vi "Nichtlinearer Beobachter.vi"(0 "x1":dbl, 1 "x3":dbl, 2 "u":dbl) -> (20 "x1_":dbl, 21 "x2_":dbl, 22 "x3_":dbl, 23 "x4_":dbl, 24 "Differenz_x1":dbl)   [LabVIEW 2014]
uses:
  Root.vi
  Root1.vi
  d(f2+g2u)_dx3.vi
  d(f2+g2u)_dx4.vi
  d(f4+g4u)_dx3.vi
  d(f4+g4u)_dx4.vi
  f2+g2u.vi
  f4+g4u.vi
  <vilib>/Simulation/Implementation/Shared/SIMSCR Execution Mode.ctl
  <vilib>/Simulation/Scripting/Companion Diagram/SimConfigNode/SimParams.ctl
  <vilib>/Simulation/Scripting/Companion Diagram/SimConfigNode/_simSolvers.ctl
  <vilib>/Simulation/Param Hierarchy/Typedefs/SIMPH Param Control Actions.ctl
  <vilib>/Simulation/Implementation/Shared/SIM limit type.ctl
  <vilib>/Simulation/Implementation/Shared/NILVSim_ParamChanged.vi
  <vilib>/Simulation/Implementation/Shared/NILVSIM_BeginStep.vi
  <vilib>/Simulation/SignalArithmetic/Implementation/NILVSim Gain.llb/SIM Gain (scalar).vi
  <vilib>/Simulation/SignalDisplay/Implementation/NILVSim Time Waveform.llb/SIM Time Waveform (vector).vi
  <vilib>/Simulation/SignalDisplay/Implementation/NILVSim Time Waveform.llb/SIM Time Waveform (scalar).vi
  <vilib>/Simulation/Nonlinear/Implementation/NILVSim Saturation.llb/SIM Saturation (scalar).vi
  <vilib>/Simulation/ContinuousLinear/Implementation/NILVSim Integrator new.llb/SIM Integrator distributor (scalar).vi
  <vilib>/Simulation/ContinuousLinear/Implementation/NILVSim Integrator new.llb/SIM Integrator collector (scalar).vi
  <vilib>/Simulation/Implementation/Shared/NILVSim_Manager.vi
  <vilib>/Utility/error.llb/Clear Errors.vi
  <vilib>/Simulation/Implementation/Shared/NILVSim_FinalizeModel.vi
  <vilib>/Simulation/Implementation/Shared/SIM Unbundle Sim Info.vi
  <vilib>/Simulation/Implementation/Shared/SIMSH Read Queue.vi
  f24.vi
  f44.vi
  f23.vi
  x3_.vi
  diff_x3.vi
  L32.vi
  diff_x1.vi
  L31.vi
  L42.vi
  L41.vi
  L11.vi
  L21.vi
  F.vi
  x4_.vi
  f43.vi
  <vilib>/Simulation/Implementation/Shared/NILVSim_Initialize.vi
  <vilib>/Simulation/Utility/Implementation/NILVSim Get Time and IsAcceptedStep.vi
  <vilib>/Simulation/Implementation/Shared/NILVSim_GetModelError.vi
  <vilib>/Simulation/Implementation/Shared/SIM SimErrorHandler.vi
  <vilib>/Simulation/Implementation/Shared/SIM Bundle Sim Info.vi
  <vilib>/Simulation/Scripting/Companion Diagram/SimConfigNode/SimDog.xnode
  <vilib>/Simulation/Implementation/XNodeFramework/SimXNode/SimX.xnode
  <vilib>/Simulation/ContinuousLinear/Implementation/NILVSim Integrator new.llb/SIM Integrator (scalar).vi
  <vilib>/Simulation/Implementation/Shared/NI_SIM_Implementation.lvlib
panel:
  out "Scope9":waveform(dbl)[](graph)
  out "Scope8":waveform(dbl)(graph)
  out "Scope7":waveform(dbl)(graph)
  out "Scope6":waveform(dbl)[](graph)
  out "Scope5":waveform(dbl)(graph)
  out "Scope4":waveform(dbl)[](graph)
  out "Scope3":waveform(dbl)[](graph)
  out "Scope2":waveform(dbl)(graph)
  out "Scope1":waveform(dbl)(graph)
  out "Scope":waveform(dbl)(graph)
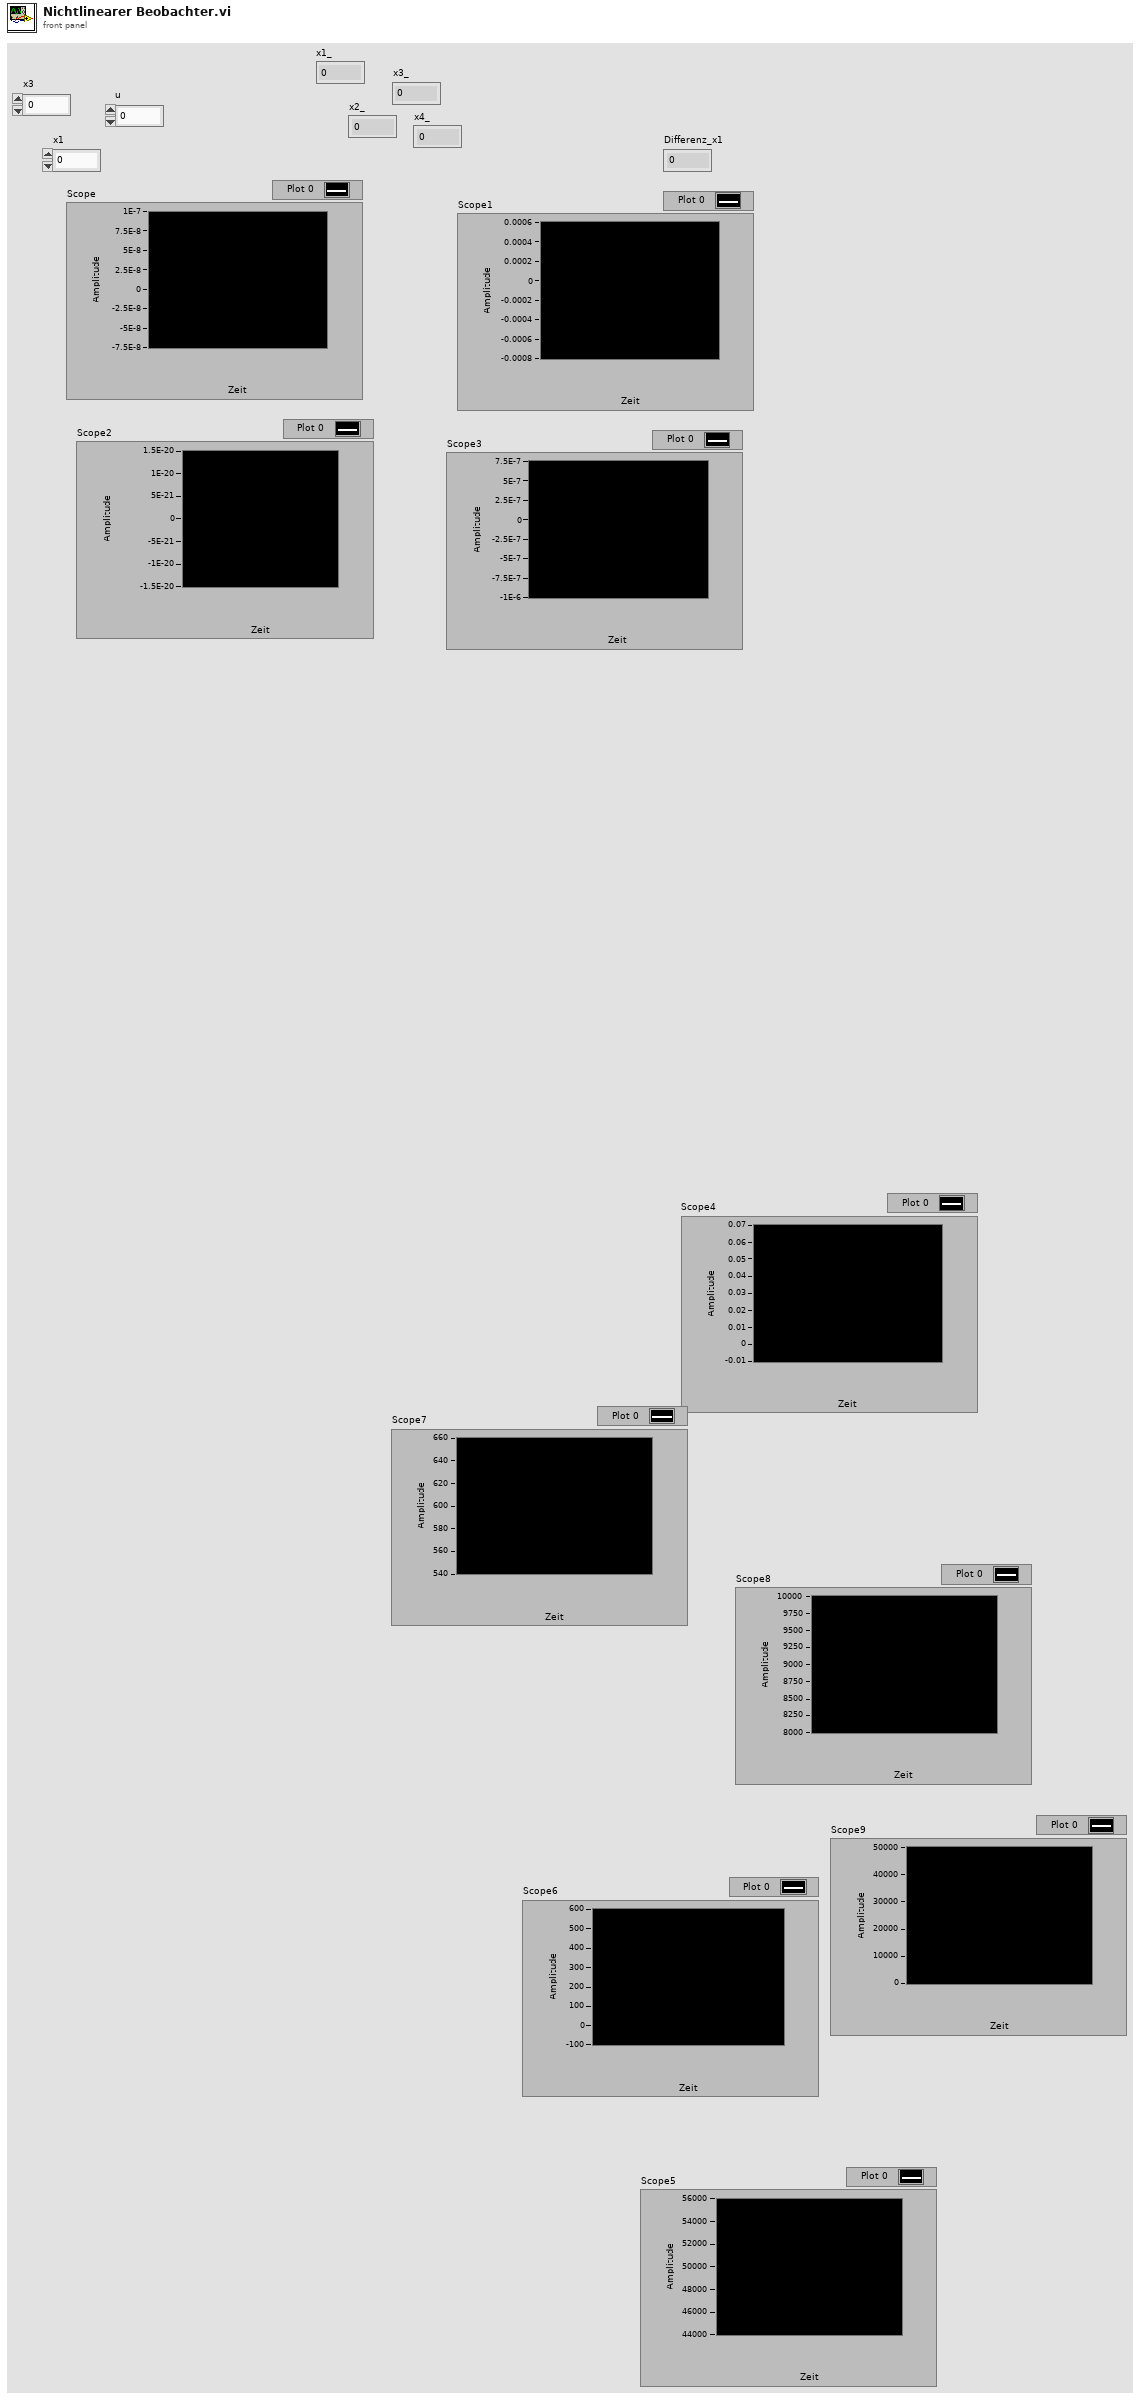
[diagram p1: front panel]
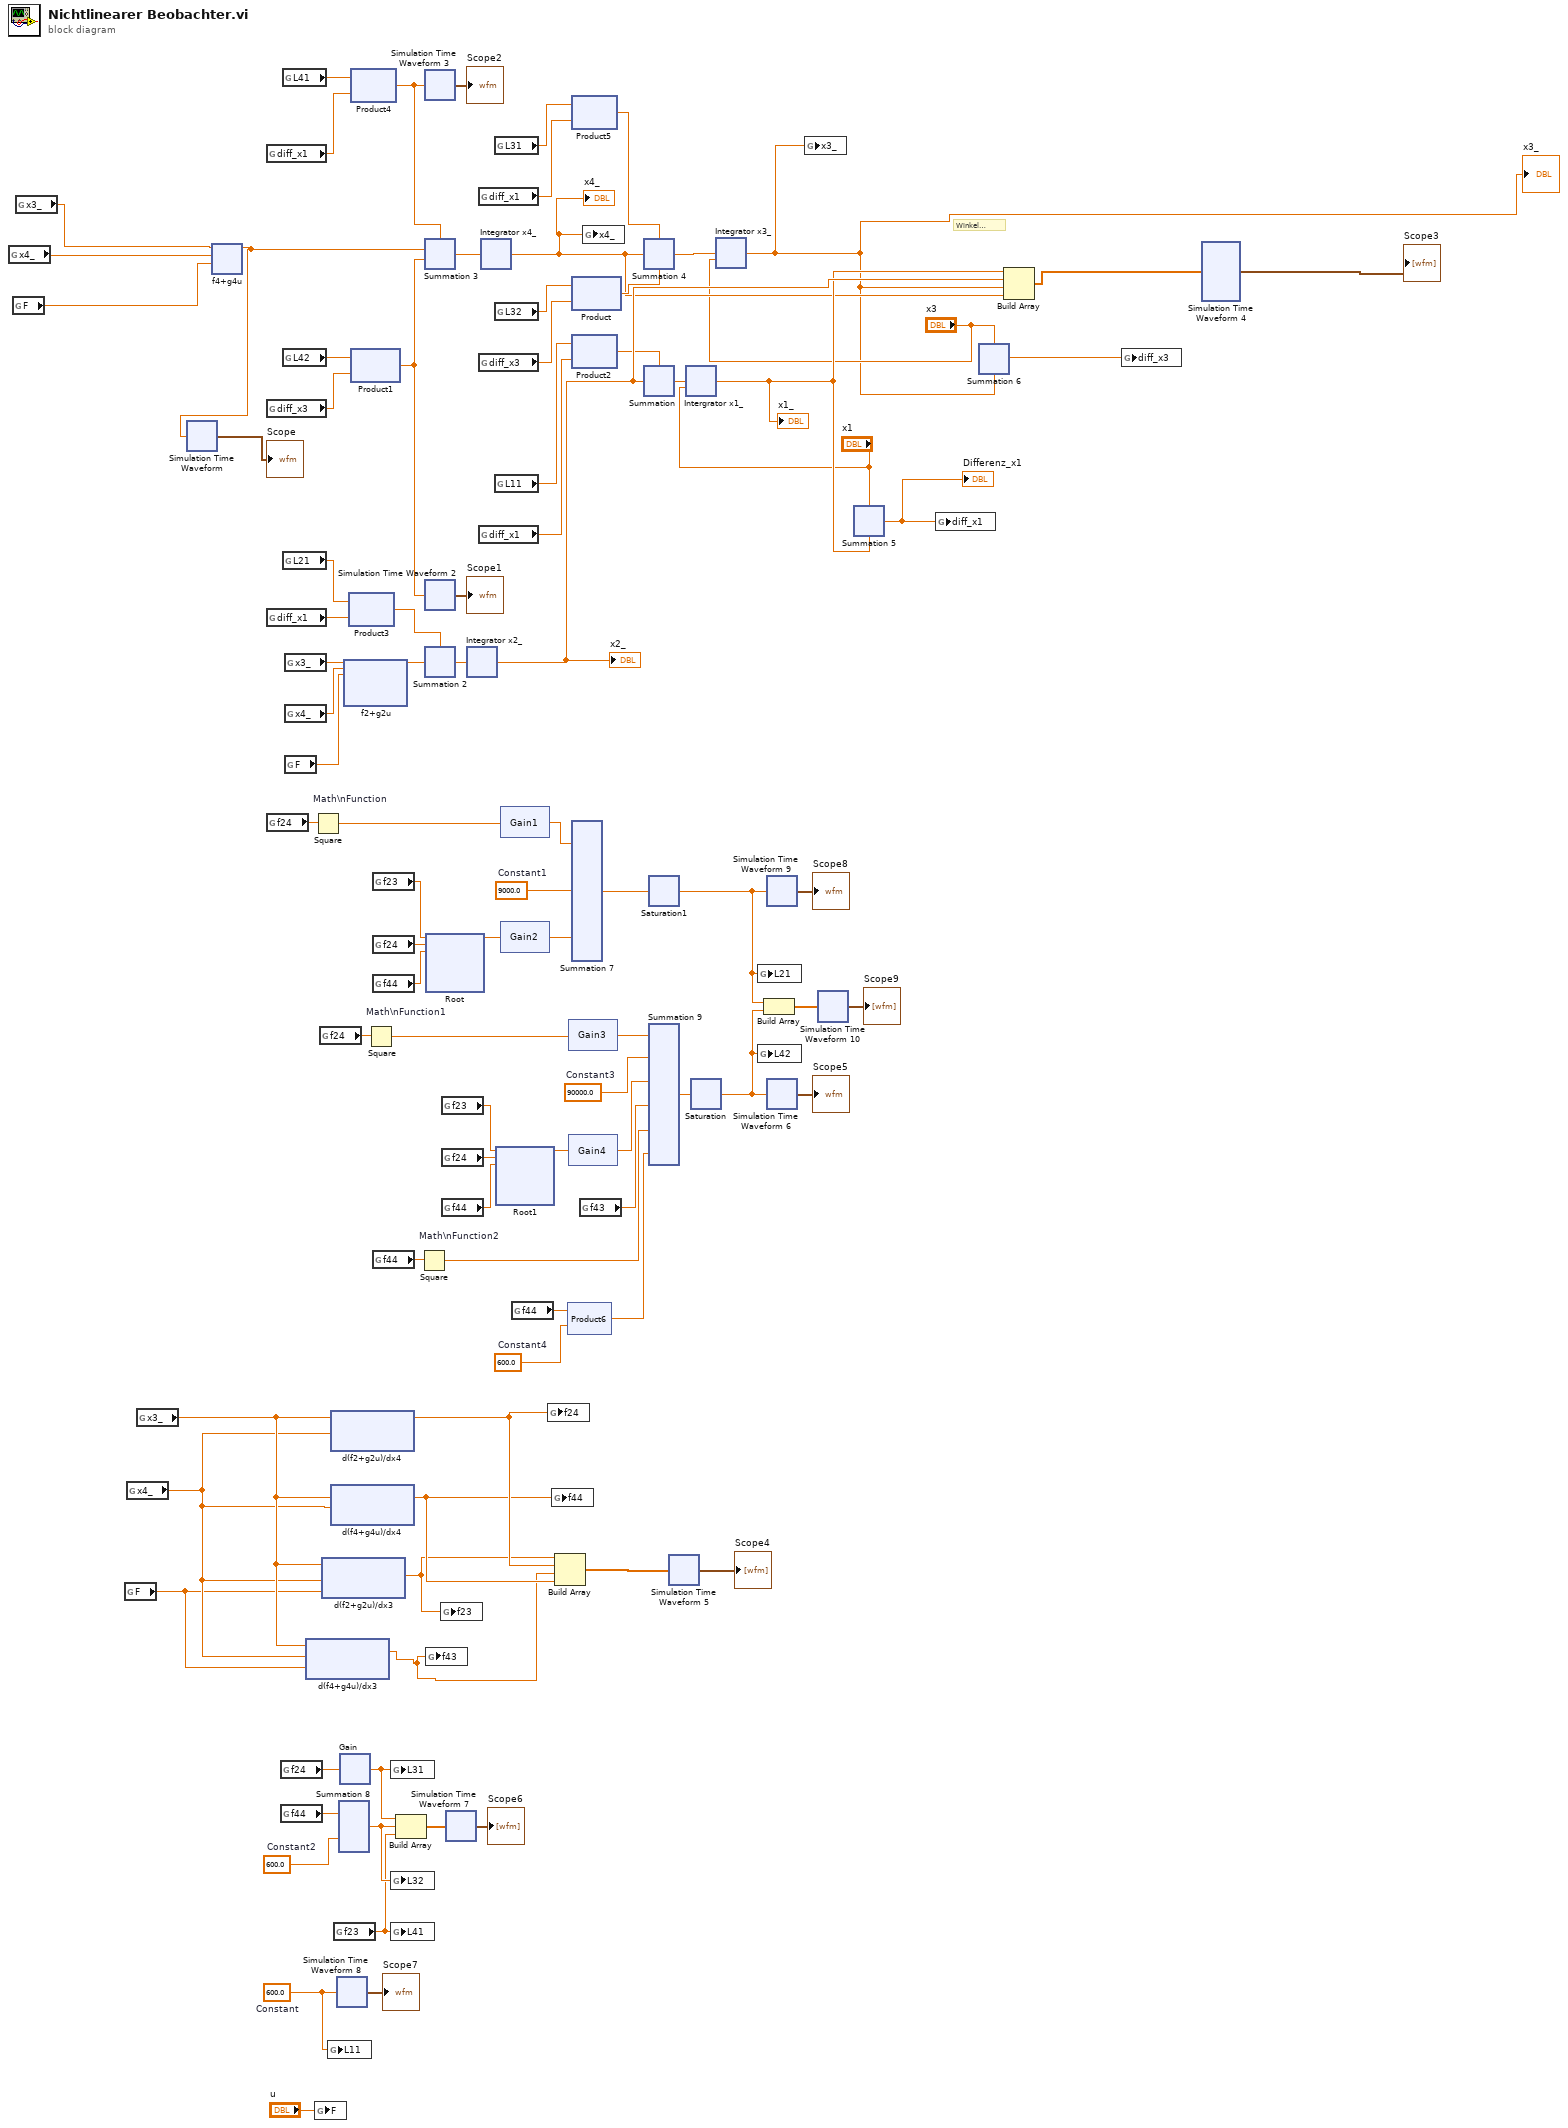
[diagram p0: block diagram]
diagram:
  w37 = 600.0  # Constant4
  w45 = 90000.0  # Constant3
  w49 = 600.0  # Constant2
  w58 = 9000.0  # Constant1
  w64 = 600.0  # Constant
  # "Winkel modulo"
  n1 = global read "x4_.vi" "x4_"() -> (w14:dbl)
  n2 = global read "From18" "F"() -> (w13:dbl)
  n3 = global read "From16" "x3_"() -> (w15:dbl)
  n4 = global read "From2" "F"() -> (w4:dbl)
  n5 = global read "From1" "x4_"() -> (w5:dbl)
  n6 = global read "From38" "x3_"() -> (w6:dbl)
  n7 = xnode "f4+g4u"("u"=w13, "x4_"=w14, "x3_"=w15) -> ("f4+g4u 2"=w12:dbl)  [unwired: 8 out]
  n8 = xnode ("Simulation Time Waveform")("Value"=w12) -> ("Waveform Chart"=→"Scope":waveform(dbl))  [unwired: 1 in]
  n9 = global read "From27" "diff_x1"() -> (w31:dbl)
  n10 = global read "From29" "diff_x3"() -> (w30:dbl)
  n11 = global read "From22" "diff_x1"() -> (w33:dbl)
  n12 = global read "From4" "f24"() -> (w61:dbl)
  n13 = global read "From3" "f24"() -> (w63:dbl)
  n14 = global read "From8" "f44"() -> (w50:dbl)
  n15 = global read "From26" "L41"() -> (w66:dbl)
  n16 = global read "From28" "L42"() -> (w65:dbl)
  n17 = global read "From23" "L21"() -> (w68:dbl)
  n18 = global read "From19" "x3_"() -> (w21:dbl)
  n19 = global read "From20" "x4_"() -> (w35:dbl)
  n20 = global read "From21" "F"() -> (w34:dbl)
  n21 = xnode "d(f4+g4u)/dx3"("x3_"=w6, "x4_"=w5, "F"=w4) -> ("d(f4+g4u)/dx3"=w7:dbl)  [unwired: 24 out]
  n22 = Square "Math\\nFunction"(x=w61) -> (x^2=w60:dbl)
  n23 = global write "Goto14" "F"("u") -> ()
  n24 = global read "From9" "f24"() -> (w48:dbl)
  n25 = xnode "d(f2+g2u)/dx3"("x3_"=w6, "x4_"=w5, "F"=w4) -> ("d(f2+g2u)/dx3"=w8:dbl)  [unwired: 24 out]
  n26 = global write "Goto1" "L11"(w64) -> ()
  n27 = xnode "d(f2+g2u)/dx4"("x3_"=w6, "x4_"=w5) -> ("d(f2+g2u)/dx4"=w10:dbl)  [unwired: 25 out]
  n28 = xnode "d(f4+g4u)/dx4"("x3_"=w6, "x4_"=w5) -> ("d(f4+g4u)/dx4"=w9:dbl)  [unwired: 25 out]
  n29 = global read "From34" "f23"() -> (w25:dbl)
  n30 = xnode ("Simulation Time Waveform 8")("Value"=w64) -> ("Waveform Chart"=→"Scope7":waveform(dbl))  [unwired: 1 in]
  n31 = xnode ("Summation 8")("Operand1"=w50, "Operand2"=w49) -> ("Result"=w51:dbl)
  n32 = xnode "Gain"("input"=w63) -> ("output"=w62:dbl)  [unwired: 3 in]
  n33 = xnode "f2+g2u"("x3_"=w21, "x4_"=w35, "u"=w34) -> ("f2+g2u"=w73:dbl)  [unwired: 24 out]
  n34 = xnode "Product3"("Operand1"=w68, "Operand2"=w33) -> ("Result"=w78:dbl)
  n35 = xnode "Product4"("Operand1"=w66, "Operand2"=w31) -> ("Result"=w71:dbl)
  n36 = xnode "Product1"("Operand1"=w65, "Operand2"=w30) -> ("Result"=w22:dbl)
  n37 = Square "Math\\nFunction1"(x=w48) -> (x^2=w47:dbl)
  n38 = global read "From6" "f23"() -> (w55:dbl)
  n39 = global read "From5" "f24"() -> (w54:dbl)
  n40 = global read "From7" "f44"() -> (w53:dbl)
  n41 = global read "From14" "f44"() -> (w40:dbl)
  n42 = global write "Goto2" "L31"(w62) -> ()
  n43 = global write "Goto8" "L32"(w51) -> ()
  n44 = global write "Goto10" "L41"(w25) -> ()
  n45 = Build Array ("Array erstellen 3")(w62, w51, w25) -> (w88:dbl[])
  n46 = Square "Math\\nFunction2"(x=w40) -> (x^2=w39:dbl)
  n47 = xnode ("Simulation Time Waveform 3")("Value"=w71) -> ("Waveform Chart"=→"Scope2":waveform(dbl))  [unwired: 1 in]
  n48 = xnode ("Summation 3")("Operand1"=w71, "Operand2"=w12, "Operand3"=w22) -> ("Result"=w77:dbl)
  n49 = xnode ("Simulation Time Waveform 2")("Value"=w22) -> ("Waveform Chart"=→"Scope1":waveform(dbl))  [unwired: 1 in]
  n50 = xnode ("Summation 2")("Operand1"=w78, "Operand2"=w73) -> ("Result"=w76:dbl)
  n51 = xnode "Root"("f23"=w55, "f24"=w54, "f44"=w53) -> ("Root"=w56:dbl)  [unwired: 24 out]
  n52 = global write "Goto5" "f43"(w7) -> ()
  n53 = global write "Goto3" "f23"(w8) -> ()
  n54 = global read "From11" "f23"() -> (w43:dbl)
  n55 = global read "From10" "f24"() -> (w42:dbl)
  n56 = global read "From12" "f44"() -> (w41:dbl)
  n57 = xnode ("Simulation Time Waveform 7")("Value"=w88) -> ("Waveform Chart"=→"Scope6":waveform(dbl)[])  [unwired: 1 in]
  n58 = xnode "Integrator x2_"("input"=w76) -> ("output"=w83:dbl)  [unwired: 9 in, 2 out]
  "x2_" <- w83
  n59 = global read "From31" "diff_x1"() -> (w29:dbl)
  n60 = global read "From33" "diff_x3"() -> (w27:dbl)
  n61 = global read "From25" "diff_x1"() -> (w32:dbl)
  n62 = xnode "Integrator x4_"("input"=w77) -> ("output"=w17:dbl)  [unwired: 9 in, 2 out]
  "x4_" <- w17
  n63 = global read "From30" "L31"() -> (w67:dbl)
  n64 = global read "From32" "L32"() -> (w28:dbl)
  n65 = global read "From24" "L11"() -> (w69:dbl)
  n66 = xnode "Root1"("f23"=w43, "f24"=w42, "f44"=w41) -> ("Root"=w44:dbl)  [unwired: 24 out]
  n67 = xnode "Gain1"("input"=w60) -> ("output"=w59:dbl)  [unwired: 3 in]
  n68 = xnode "Gain2"("input"=w56) -> ("output"=w57:dbl)  [unwired: 3 in]
  n69 = global read "From15" "f44"() -> (w38:dbl)
  n70 = global write "Goto4" "f24"(w10) -> ()
  n71 = global write "Goto6" "f44"(w9) -> ()
  n72 = Build Array ("Array erstellen 2")(w8, w10, w7, w9) -> (w11:dbl[])
  n73 = xnode "Product6"("Operand1"=w38, "Operand2"=w37) -> ("Result"=w36:dbl)
  n74 = xnode "Gain3"("input"=w47) -> ("output"=w46:dbl)  [unwired: 3 in]
  n75 = xnode "Gain4"("input"=w44) -> ("output"=w23:dbl)  [unwired: 3 in]
  n76 = xnode "Product5"("Operand1"=w67, "Operand2"=w29) -> ("Result"=w70:dbl)
  n77 = xnode "Product"("Operand1"=w28, "Operand2"=w27) -> ("Result"=w26:dbl)
  n78 = xnode "Product2"("Operand1"=w69, "Operand2"=w32) -> ("Result"=w79:dbl)
  n79 = xnode ("Summation 7")("Operand1"=w59, "Operand2"=w58, "Operand3"=w57) -> ("Result"=w52:dbl)
  n80 = global read "From13" "f43"() -> (w24:dbl)
  n81 = global write "Goto13" "x4_"(w17) -> ()
  n82 = xnode ("Summation 4")("Operand1"=w70, "Operand2"=w17, "Operand3"=w26) -> ("Result"=w81:dbl)
  n83 = xnode ("Summation")("Operand1"=w79, "Operand2"=w83) -> ("Result"=w82:dbl)
  n84 = xnode "Saturation1"("input"=w52) -> ("output"=w18:dbl)  [unwired: 4 in]
  n85 = xnode ("Summation 9")("Operand1"=w46, "Operand2"=w45, "Operand3"=w23, "Operand4"=w24, "Operand5"=w39, "Operand6"=w36) -> ("Result"=w20:dbl)
  n86 = xnode ("Simulation Time Waveform 5")("Value"=w11) -> ("Waveform Chart"=→"Scope4":waveform(dbl)[])  [unwired: 1 in]
  n87 = xnode "Intergrator x1_"("input"=w82, "initial condition"="x1") -> ("output"=w80:dbl)  [unwired: 8 in, 2 out]
  "x1_" <- w80
  n88 = xnode "Saturation"("input"=w20) -> ("output"=w19:dbl)  [unwired: 4 in]
  n89 = xnode "Integrator x3_"("input"=w81, "initial condition"="x3") -> ("output"=w2:dbl)  [unwired: 8 in, 2 out]
  "x3_" <- w2
  n90 = global write "Goto7" "L21"(w18) -> ()
  n91 = global write "Goto9" "L42"(w19) -> ()
  n92 = Build Array ("Array erstellen 4")(w18, w19) -> (w84:dbl[])
  n93 = xnode ("Simulation Time Waveform 9")("Value"=w18) -> ("Waveform Chart"=→"Scope8":waveform(dbl))  [unwired: 1 in]
  n94 = xnode ("Simulation Time Waveform 6")("Value"=w19) -> ("Waveform Chart"=→"Scope5":waveform(dbl))  [unwired: 1 in]
  n95 = global write "Goto12" "x3_"(w2) -> ()
  n96 = xnode ("Simulation Time Waveform 10")("Value"=w84) -> ("Waveform Chart"=→"Scope9":waveform(dbl)[])  [unwired: 1 in]
  n97 = xnode ("Summation 5")("Operand1"="x1", "Operand2"=w80) -> ("Result"=w75:dbl)
  "Differenz_x1" <- w75
  n98 = global write "Goto15" "diff_x1"(w75) -> ()
  n99 = xnode ("Summation 6")("Operand1"="x3", "Operand2"=w2) -> ("Result"=w74:dbl)
  n100 = Build Array ("Array erstellen")(w80, w83, w2, w17) -> (w92:dbl[])
  n101 = global write "Goto16" "diff_x3"(w74) -> ()
  n102 = xnode ("Simulation Time Waveform 4")("Value"=w92) -> ("Waveform Chart"=→"Scope3":waveform(dbl)[])  [unwired: 1 in]
